vi "Set AutomaticSortEnabled.vi"(8 "error in":errorcluster, 10 "AutomaticSortEnabled":bool, 11 "ColumnHeader in":refnum<class "Column Header.lvclass">) -> (0 "error out":errorcluster, 3 "ColumnHeader out":refnum<class "Column Header.lvclass">)   [LabVIEW 2024, in "SourceGrid.lvlib" / "Column Header.lvclass"]
uses:
  Column Header.lvclass
  Cell/Cell.lvclass/Cell.ctl
  D:/git/Sourcegrid-LabVIEW/dll/SourceGrid.dll
  dll/SourceGrid.dll
  Column Header.lvclass/Column Header.ctl
  Cell/Cell.lvclass
  D:/git/Sourcegrid-LabVIEW/source/Cells/Cell/Cell.lvclass
  D:/git/Sourcegrid-LabVIEW/source/Cells/ColumnHeader/Column Header.lvclass
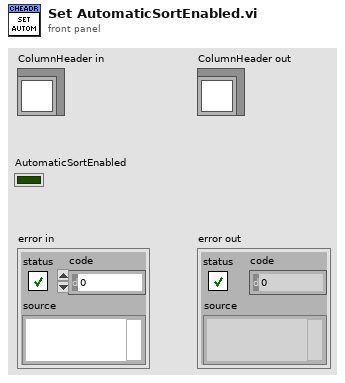
[diagram p1: front panel]
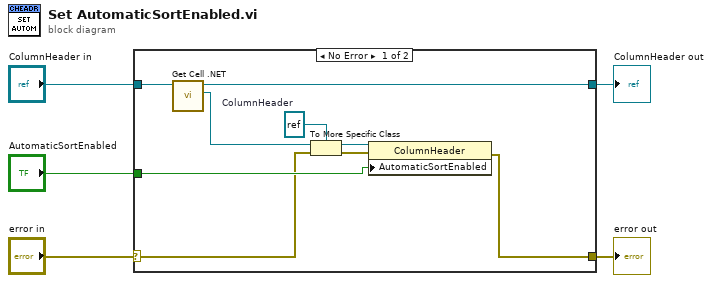
[diagram p0: block diagram]
diagram:
  n1 = case shown="No Error" "error in" {
    selector: "error in" -> [w7 w15]
    tunnel: [w12 w15] -> w4
    tunnel: [w11 w16] -> w2
    tunnel: "ColumnHeader in" -> [w13 w16]
    tunnel: "AutomaticSortEnabled" -> [w14 _]
    frame No Error {
      w8 = refnum<k24> refnum  # ColumnHeader
      n2 = call "Get Cell .NET.vi"("Cell in"=w13) -> ("Cell .NET"=w10:refnum<k24>, "Cell in"=w11:refnum<class "Column Header.lvclass">)  [unwired: 9 in]
      n3 = To More Specific Class(target class=w8, reference=w10, error in=w7) -> (specific class reference=w9:refnum<k24>, error out=w6:errorcluster)
      n4 = property class="ColumnHeader"(reference=w9, error in=w6, "AutomaticSortEnabled"=w14) -> (error out=w12:errorcluster)  [unwired: 1 out]
    }
    frame Error {
    }
  }
  "error out" <- w4
  "ColumnHeader out" <- w2
